vi "Prepare_For_Consolidated_Save.vi"(7 "inside target file":bool, 8 "error in (no error)":errorcluster, 11 "AB_Source in":refnum<class "AB_Source.lvclass">) -> (0 "error out":errorcluster, 2 "item_Data":T1, 3 "AB_Source out":refnum<class "AB_Source.lvclass">)   [LabVIEW 2020, in "AB_Source.lvclass"]
uses:
  <vilib>/AppBuilder/AB_Classes/Source/AB_Source.lvclass
  <vilib>/AppBuilder/Engine/AB_Engine_Consolidated_Save_Item_Info.ctl
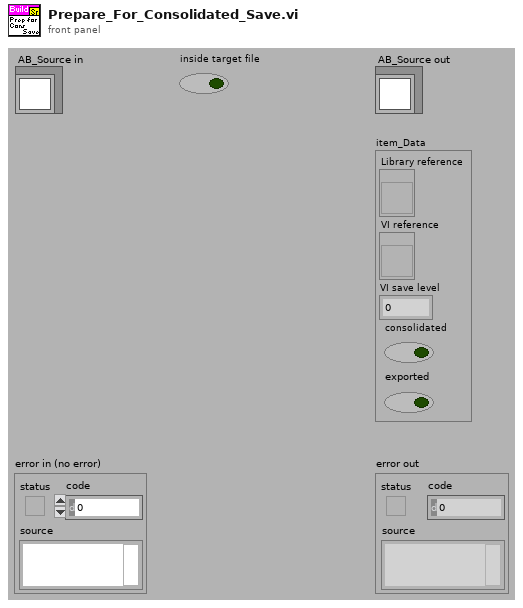
[diagram p1: front panel]
types:
  T1 = typedef "AB_Engine_Consolidated_Save_Item_Info.ctl" = cluster{"Library reference":refnum<vi>, "VI reference":refnum<vi>, "VI save level":i32, "consolidated":bool, "exported":bool}
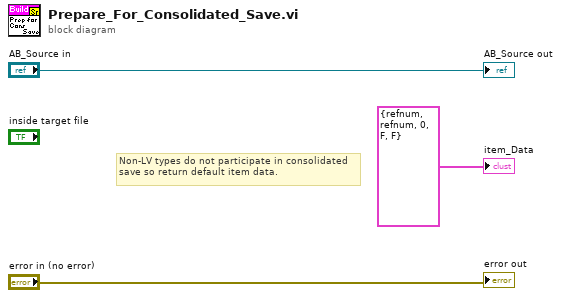
[diagram p0: block diagram]
diagram:
  # "Non-LV types do not participate in consolidated save so return default item data."
  "error out" <- "error in (no error)"
  "AB_Source out" <- "AB_Source in"
  "item_Data" <- T1 {"Library reference"=refnum, "VI reference"=refnum, "VI save level"=0, "consolidated"=FALSE, "exported"=FALSE} ("item_Data")
